vi "Excel_Quit_Graph.vi"(0 "Excel._Worksheet":refnum<k7>, 5 "Shapes":refnum<k7>, 9 "Chart index":i16=-1, 11 "error in (no error)":errorcluster) -> (15 "error out":errorcluster)   [LabVIEW 2017, in "NI_ReportGenerationToolkit.lvlib"]
uses:
  <vilib>/addons/_office/NI_ReportGenerationToolkit.lvlib
panel:
  in  "Excel._OLEObject":refnum<k7>
  in  "Graph.Chart":refnum<k7>
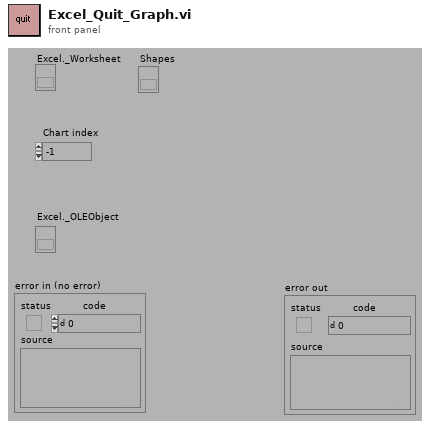
[diagram p1: front panel]
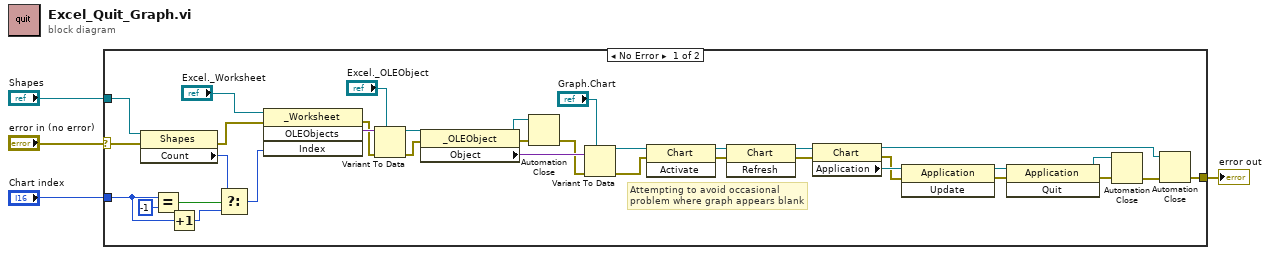
[diagram p0: block diagram]
diagram:
  n1 = case shown="No Error" "error in (no error)" {
    selector: "error in (no error)" -> [w6 w40]
    tunnel: "Chart index" -> [w28 _]
    tunnel: [w22 w40] -> w3
    tunnel: "Shapes" -> [w7 _]
    frame No Error {
      # "Attempting to avoid occasional problem where graph appears blank"
      n2 = property class="Shapes"(reference=w7, error in=w6) -> (error out=w31:errorcluster, "Count"=w30:i32)  [unwired: 1 out]
      n3 = Equal?(x=w28, y=i16 -1) -> (x = y?=w39:bool)
      n4 = Increment(x=w28) -> (x+1=w37:i16)
      n5 = Select(t=w30, s=w39, f=w37) -> (s? t:f=w29:i32)
      n6 = invoke class="_Worksheet" method="OLEObjects"(reference="Excel._Worksheet", error in=w31, "Index"=w29) -> (error out=w34:errorcluster, "OLEObjects"=w35:variant)  [unwired: 1 in, 2 out]
      n7 = Variant To Data(error in=w34, type="Excel._OLEObject", Variant=w35) -> (data=w18:refnum<k7>, error out=w25:errorcluster)
      n8 = property class="_OLEObject"(reference=w18, error in=w25) -> (reference out=w32:refnum<k7>, error out=w33:errorcluster, "Object"=w27:variant)
      n9 = Automation Close(3:w33, 5:w32) -> (0:w26:errorcluster)
      n10 = Variant To Data(error in=w26, type="Graph.Chart", Variant=w27) -> (data=w16:refnum<k7>, error out=w15:errorcluster)
      n11 = invoke class="Chart" method="Activate"(reference=w16, error in=w15) -> (reference out=w9:refnum<k7>, error out=w11:errorcluster)  [unwired: 1 in, 1 out]
      n12 = invoke class="Chart" method="Refresh"(reference=w9, error in=w11) -> (reference out=w8:refnum<k7>, error out=w10:errorcluster)  [unwired: 1 in, 1 out]
      n13 = property class="Chart"(reference=w8, error in=w10) -> (reference out=w13:refnum<k7>, error out=w20:errorcluster, "Application"=w21:refnum<k7>)
      n14 = invoke class="Application" method="Update"(reference=w21, error in=w20) -> (reference out=w19:refnum<k7>, error out=w12:errorcluster)  [unwired: 1 in, 1 out]
      n15 = invoke class="Application" method="Quit"(reference=w19, error in=w12) -> (reference out=w23:refnum<k7>, error out=w24:errorcluster)  [unwired: 1 in, 1 out]
      n16 = Automation Close(3:w24, 5:w23) -> (0:w14:errorcluster)
      n17 = Automation Close(3:w14, 5:w13) -> (0:w22:errorcluster)
    }
    frame Error {
    }
  }
  "error out" <- w3
